vi "Throttlebrakeswitch.vi"(8 "pitch[deg]":dbl format="%#_13g", 9 "thresh":dbl=0.01 format="%#_13g", 10 "v0":dbl=8.0 format="%#_13g", 11 "vel_limit":dbl format="%#_13g") -> (0 "Verror":dbl, 3 "u":dbl)   [LabVIEW 2015]
uses:
  rio_Global.vi
panel:
  in  "an":dbl=-2.943 format="%#_13g"
  in  "ap":dbl=0.0981
  in  "dt":dbl=1.0 format="%#_13g"
  out "D":dbl=1300.0
  out "m":dbl=1300.0
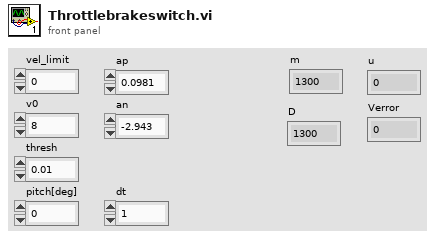
[diagram p1: front panel]
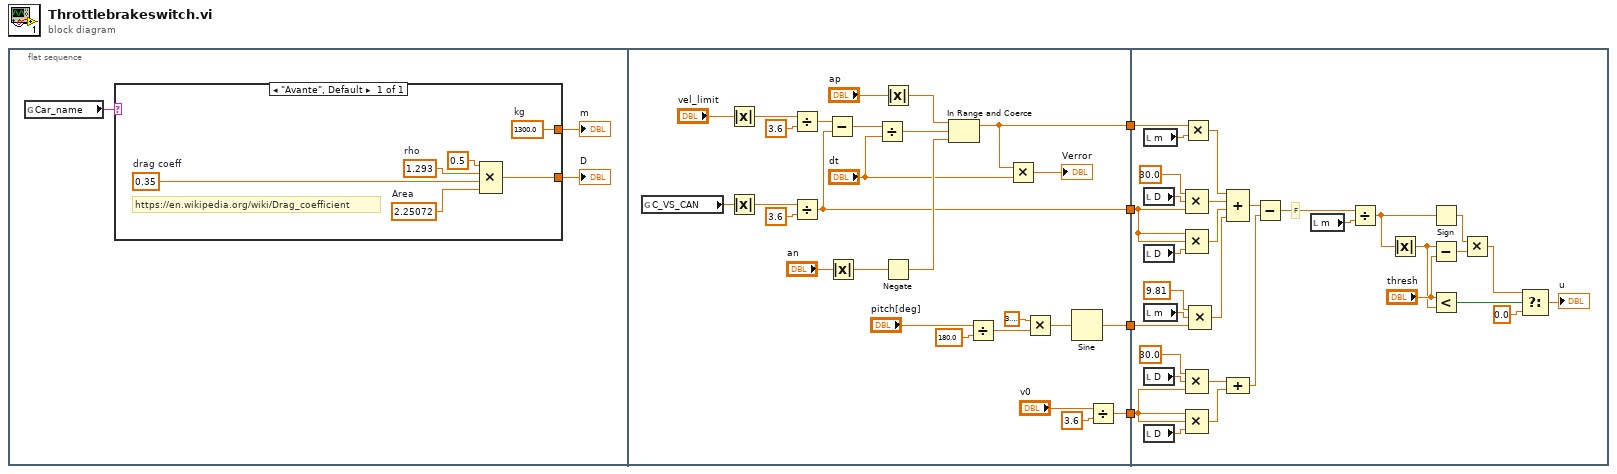
[diagram p0: block diagram]
diagram:
  n1 = flat-sequence {
    tunnel: [w25] -> w4
    tunnel: [w22] -> w3
    tunnel: [w21] -> w2
    tunnel: [w16] -> w1
    tunnel: w4 -> [w65]
    tunnel: w3 -> [w58]
    tunnel: w2 -> [w42]
    tunnel: w1 -> [w41]
    frame #0 {
      n2 = global read "rio_Global.vi" "Car_name"() -> (w7:string)
      n3 = case shown="\"Avante\", Default" w7 {
        tunnel: [w9] -> w6
        tunnel: [w8] -> w5
        frame "Avante", Default {
          w10 = 2.25072  # Area
          w11 = 0.35  # drag coeff
          w12 = 1.293  # rho
          w9 = 1300.0  # kg
          # "https://en.wikipedia.org/wiki/Drag_coefficient"
          n4 = Compound Arithmetic op=MULTIPLY(0.5 ("value"), w12, w11, w10) -> (w8:dbl)
        }
      }
      "m" <- w6
      "D" <- w5
    }
    frame #1 {
      n5 = global read "rio_Global.vi" "C_VS_CAN"() -> (w20:dbl)
      n6 = Absolute Value(x="vel_limit") -> (abs(x)=w18:dbl)
      n7 = Absolute Value(x=w20) -> (abs(x)=w19:dbl)
      n8 = Divide(x=w18, y=3.6) -> (x/y=w38:dbl)
      n9 = Divide(x=w19, y=3.6) -> (x/y=w21:dbl)
      n10 = Subtract(x=w38, y=w21) -> (x-y=w37:dbl)
      n11 = Absolute Value(x="an") -> (abs(x)=w32:dbl)
      n12 = Divide(x=w37, y="dt") -> (x/y=w36:dbl)
      n13 = Absolute Value(x="ap") -> (abs(x)=w34:dbl)
      n14 = Negate(x=w32) -> (-x=w31:dbl)
      n15 = In Range and Coerce(upper limit=w34, x=w36, lower limit=w31) -> (coerced(x)=w16:dbl)  [unwired: 1 out]
      n16 = Divide(x="pitch[deg]", y=180.0) -> (x/y=w28:dbl)
      n17 = Multiply(x=w16, y="dt") -> (x*y=→"Verror":dbl)
      n18 = Multiply(x=3.141592653589793, y=w28) -> (x*y=w26:dbl)
      n19 = Sine(x=w26) -> (sin(x)=w25:dbl)
      n20 = Divide(x="v0", y=3.6) -> (x/y=w22:dbl)
    }
    frame #2 {
      # "F"
      n21 = local read "m"() -> (w72:dbl)
      n22 = local read "D"() -> (w69:dbl)
      n23 = local read "D"() -> (w43:dbl)
      n24 = local read "m"() -> (w67:dbl)
      n25 = local read "D"() -> (w60:dbl)
      n26 = local read "D"() -> (w57:dbl)
      n27 = Multiply(x=w41, y=w72) -> (x*y=w71:dbl)
      n28 = Compound Arithmetic op=MULTIPLY(30.0 ("x"), w69, w42) -> (w68:dbl)
      n29 = Compound Arithmetic op=MULTIPLY(w42, w42, w43) -> (w64:dbl)
      n30 = Compound Arithmetic op=MULTIPLY(30.0 ("x"), w60, w58) -> (w61:dbl)
      n31 = Compound Arithmetic op=MULTIPLY(w58, w58, w57) -> (w62:dbl)
      n32 = Compound Arithmetic op=MULTIPLY(9.81 ("x"), w67, w65) -> (w63:dbl)
      n33 = Compound Arithmetic op=ADD(w71, w68, w64, w63) -> (w56:dbl)
      n34 = Compound Arithmetic op=ADD(w61, w62) -> (w55:dbl)
      n35 = Subtract(x=w56, y=w55) -> (x-y=w53:dbl)
      n36 = local read "m"() -> (w54:dbl)
      n37 = Divide(x=w53, y=w54) -> (x/y=w50:dbl)
      n38 = Absolute Value(x=w50) -> (abs(x)=w45:dbl)
      n39 = Sign(1:w50) -> (0:w49:dbl)
      n40 = Subtract(x=w45, y="thresh") -> (x-y=w51:dbl)
      n41 = Less?(x="thresh", y=w45) -> (x < y?=w52:bool)
      n42 = Multiply(x=w49, y=w51) -> (x*y=w48:dbl)
      n43 = Select(t=w48, s=w52, f=0.0) -> (s? t:f=→"u":dbl)
    }
  }
